vi "UpdateClassTemplate.vi"(0 "ClassWriterGOOP300In":refnum<class "ClassWriterGOOP400.lvclass">, 1 "LVClassLibraryRef":refnum<vi>, 2 "ProgressBar":refnum<vi>, 5 "error in (no error)":errorcluster) -> (14 "ClassWriterGOOP300Out":refnum<class "ClassWriterGOOP400.lvclass">, 19 "error out":errorcluster)   [LabVIEW 2020, in "ClassWriterGOOP400.lvclass"]
uses:
  <resource>/Framework/Providers/Open_GDS/ClassProviders/Provider_EndevoGOOP400/ClassWriterGOOP400_class/ClassWriterGOOP400.lvclass
  <resource>/Framework/Providers/Open_GDS/ClassProviders/Provider_LvNativeClass/ClassWriterNative_class/ClassWriterNative.lvclass
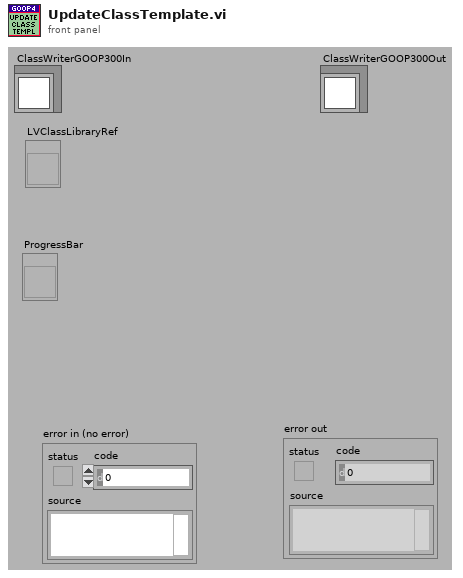
[diagram p1: front panel]
types:
  T1 = cluster{"VIs":refnum<vi>[], "VIRelPath":path[], "Application":refnum<vi>, "TemplateVersions":string, "Create":refnum<vi>, "NewVIIdx":i32, "PersistentExists":bool, "PersistentNewVersion":bool}
  T2 = enum32{"invalid lock state", "Not Locked", "Locked (No Password)", "Password-protected"}
  T3 = enum16{"Share clones between instances", "Preallocate clone for each instance"}
  T4 = typedef "GDSLvCLass_ClassSettingsType.ctl" = cluster{"ClassProviderName":string, "ClassTemplateUsed":string, "ClassTemplateVersion":string, "ClassDescription":string, "PlugIns":T5[], "ConnectorPanePattern":string}
  T5 = typedef "GDSLvClass_PlugIn.ctl" = cluster{"Type":T6, "ID":string, "Version":string, "Path":path, "Name":string, "Data":variant}
  T6 = typedef "GDSLvClass_PlugInTypes.ctl" = enum16{"DesignPattern", "MethodTypes"}
  T7 = cluster{"ID":string, "Version":string, "PlugIn":path, "Type":string, "Name":string, "Desc":string, "Supports":cluster{"Provider":string, "Templates":string}[], "DependenciesID":string[], "OnlyOne":bool}
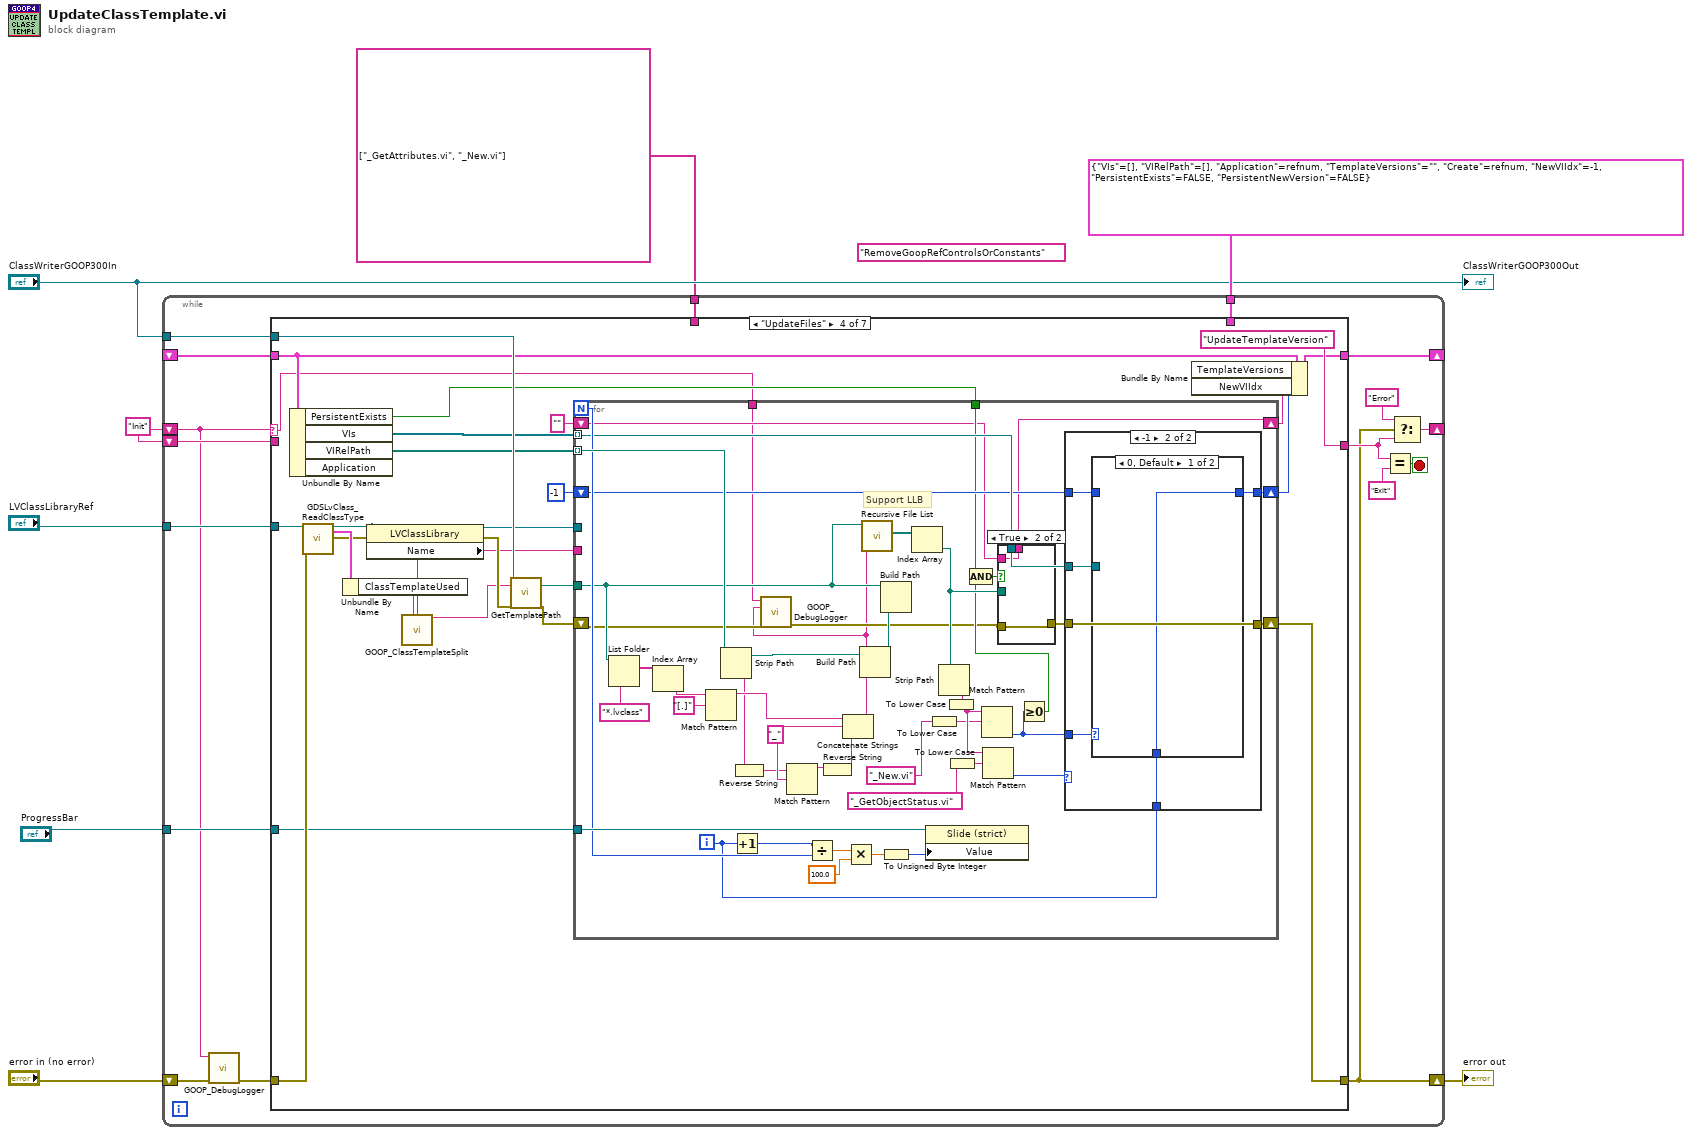
[diagram p0: block diagram]
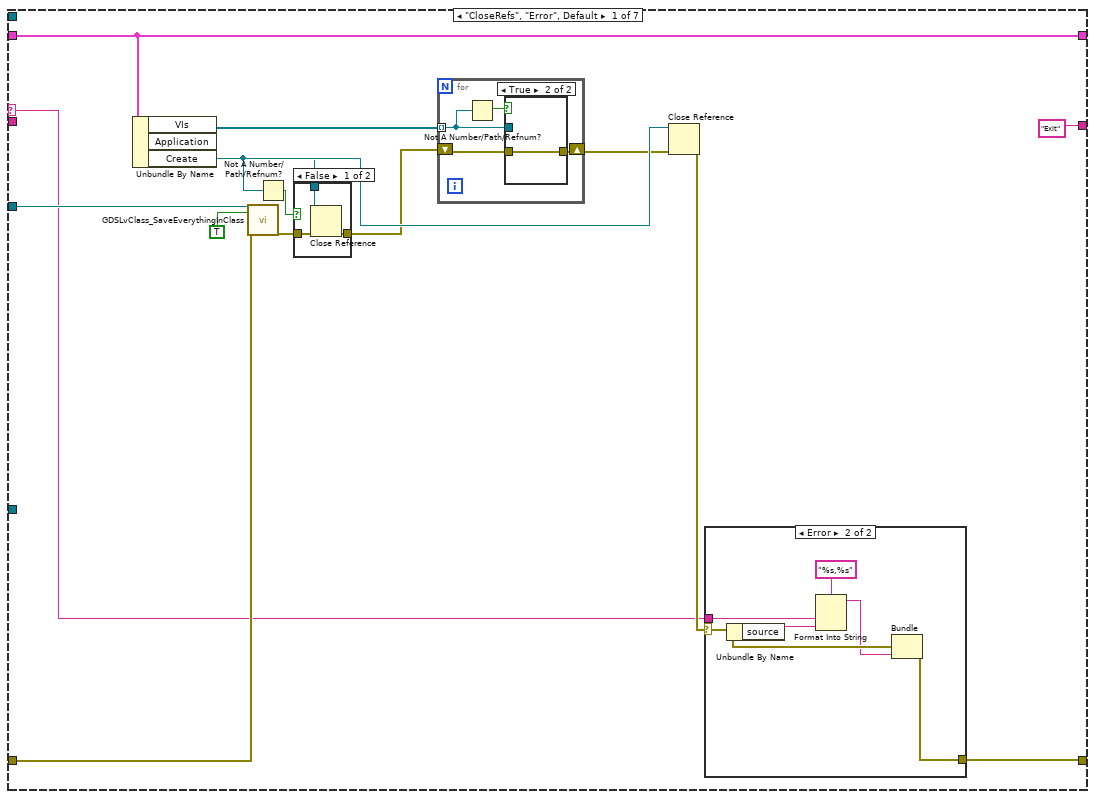
[diagram p2: hidden frame]
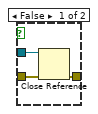
[diagram p5: hidden frame]
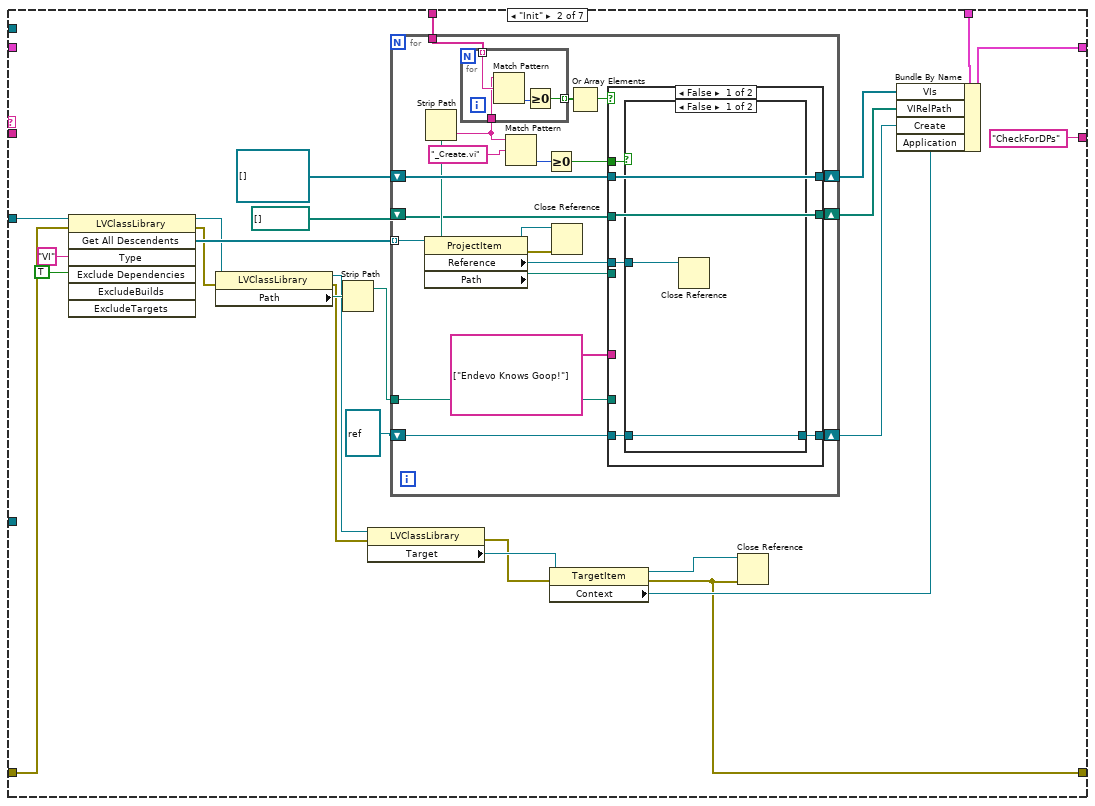
[diagram p6: hidden frame]
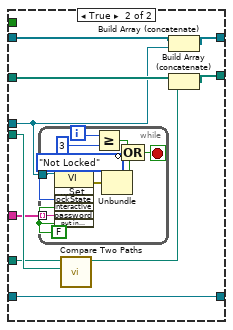
[diagram p8: hidden frame]
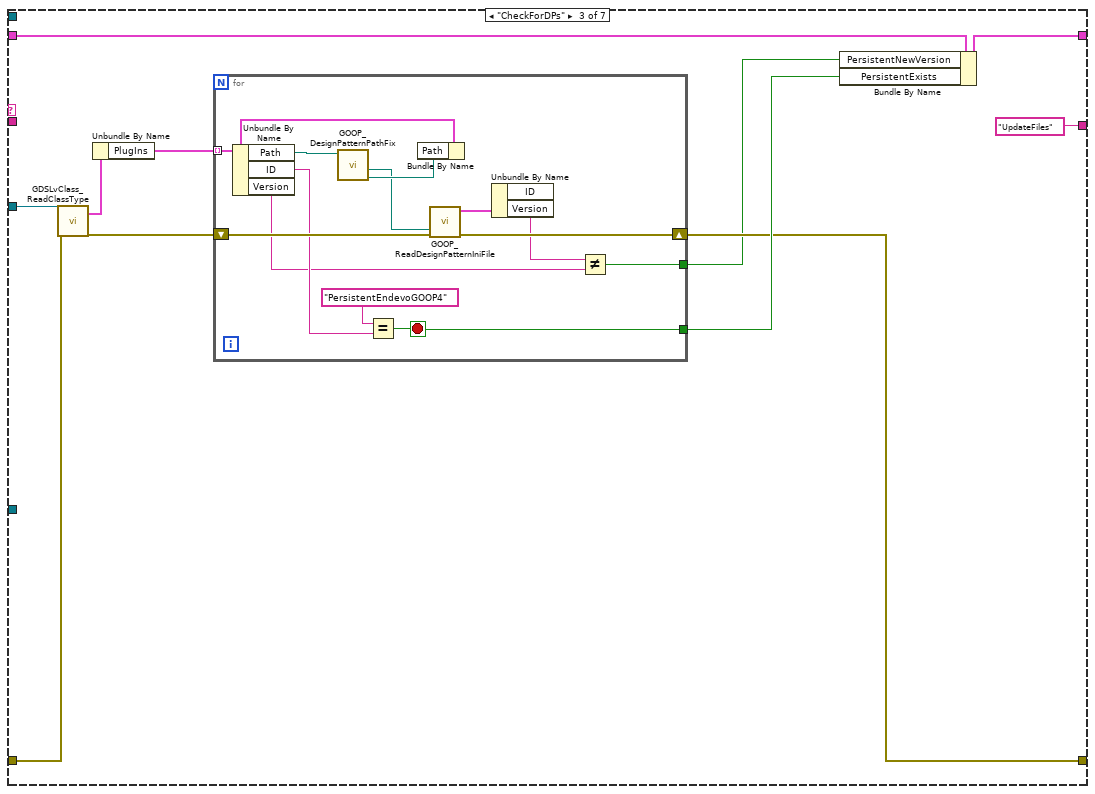
[diagram p9: hidden frame]
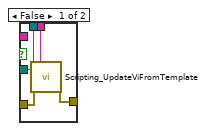
[diagram p10: hidden frame]
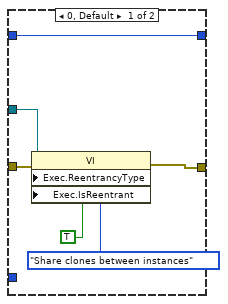
[diagram p11: hidden frame]
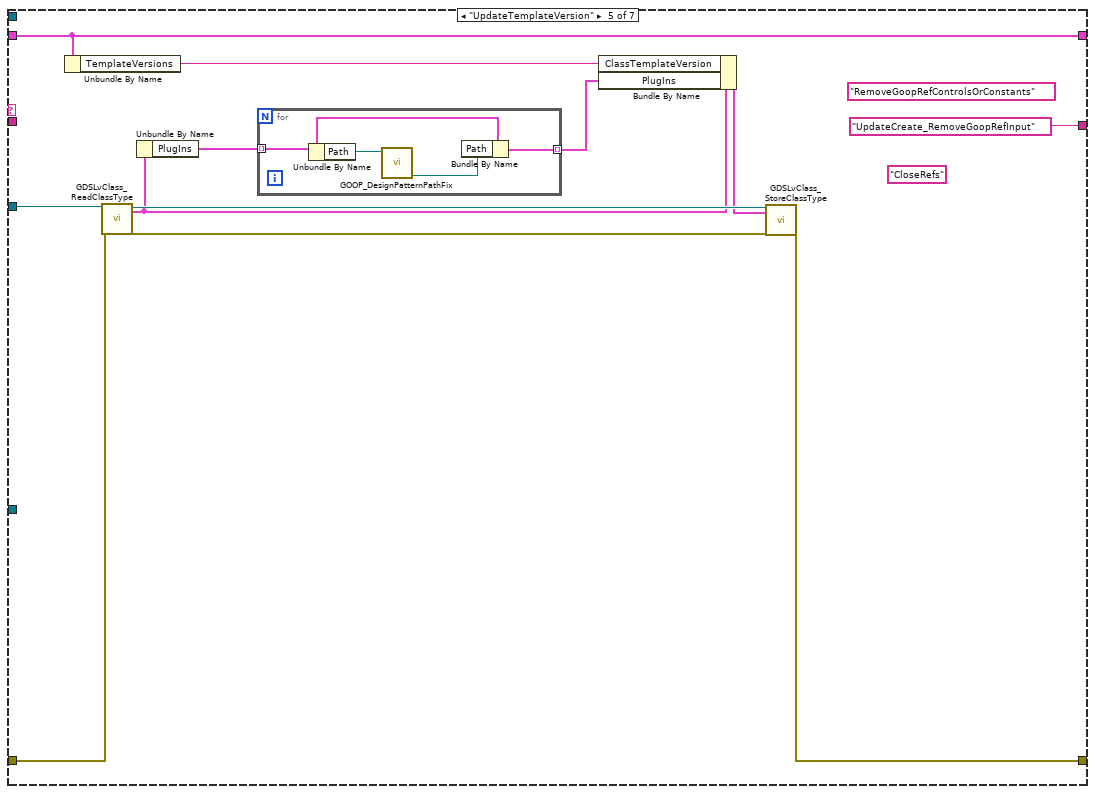
[diagram p13: hidden frame]
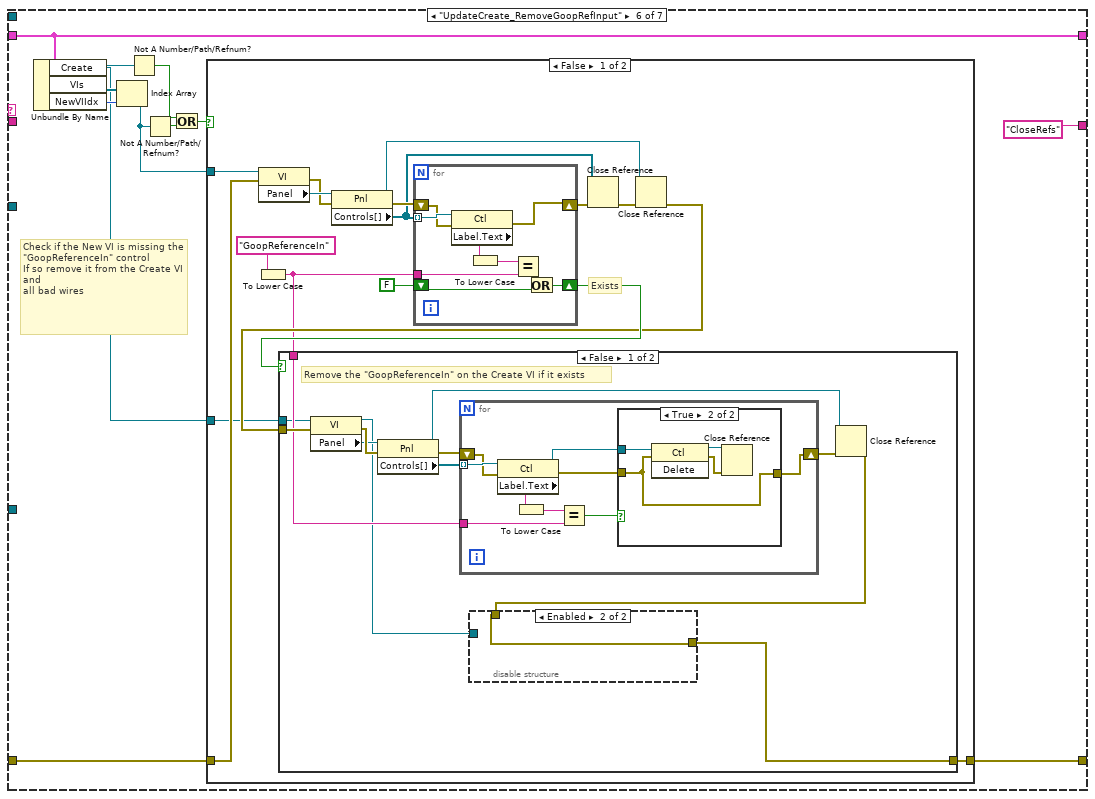
[diagram p14: hidden frame]
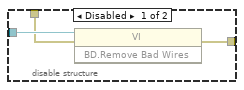
[diagram p15: hidden frame]
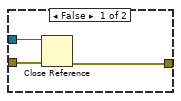
[diagram p16: hidden frame]
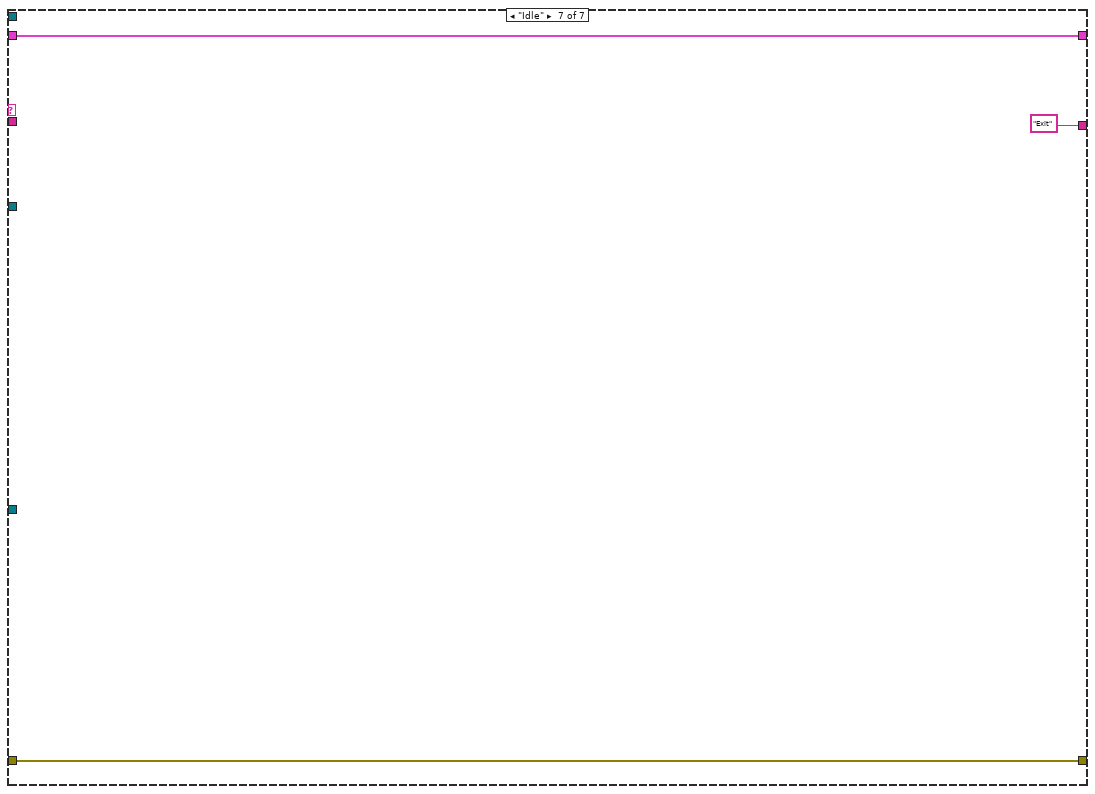
[diagram p19: hidden frame]
diagram:
  (unwired) "RemoveGoopRefControlsOrConstants"
  w1 = "Init"
  n1 = while {
    shift-right: [w20] -> w7
    shift-left: "error in (no error)" -> [w11]
    shift-right: [w25] -> _
    shift-left: w1 -> [w9]
    shift-right: [w19] -> _
    shift-left: _ -> [w18]
    tunnel: "LVClassLibraryRef" -> [w17]
    tunnel: T1 {"VIs"=[], "VIRelPath"=[], "Application"=refnum, "TemplateVersions"="", "Create"=refnum, "NewVIIdx"=-1, "PersistentExists"=FALSE, "PersistentNewVersion"=FALSE} -> [w16]
    tunnel: "ClassWriterGOOP300In" -> [w15]
    tunnel: "ProgressBar" -> [w14]
    tunnel: string[] ["_GetAttributes.vi", "_New.vi"] ("Array") -> [w13]
    shift-left: w1 -> [w12]
    stop <- w24 stop-if-true
    n2 = call <resource>:"GOOP_DebugLogger.vi"("error in (no error)"=w11, "State"=w9) -> ("error out"=w10:errorcluster)  [unwired: 7 in, 2 out]
    n3 = case shown="\"UpdateFiles\"" w9 {
      selector: w9 -> [w28 _ _ w166 _ _ _]
      tunnel: w10 -> [w34 w66 w147 w180 w261 w274 w343]
      tunnel: [w27 w61 w141 w174 w260 w273 w343] -> w20
      tunnel: ["Exit" "CheckForDPs" "UpdateFiles" "UpdateTemplateVersion" "UpdateCreate_RemoveGoopRefInput" "CloseRefs" "Exit"] -> w21
      tunnel: [w39 w85 w143 w175 w265 w280 w342] -> w19
      tunnel: w18 -> [w39 _ w139 w176 w265 w280 w342]
      tunnel: w17 -> [w35 w84 w145 w187 w264 _ _]
      tunnel: w16 -> [_ w78 _ _ _ _ _]
      tunnel: w15 -> [_ _ _ w185 _ _ _]
      tunnel: w14 -> [_ _ _ w173 _ _ _]
      tunnel: w13 -> [_ w65 _ _ _ _ _]
      tunnel: w12 -> [_ _ _ _ _ _ _]
      frame "CloseRefs", "Error", Default {
        n4 = Unbundle By Name(w39) -> ("VIs"=w38:refnum<vi>[], "Application"=w37:refnum<vi>, "Create"=w31:refnum<vi>)
        n5 = call <resource>:"GDSLvClass_SaveEverythingInClass.vi"("ClassRefIn"=w35, "ForceResaving(False)"=TRUE, "error in"=w34) -> ("error out"=w33:errorcluster)  [unwired: 15 in, 1 out]
        n6 = Not A Number/Path/Refnum?(number/path/refnum=w31) -> (NaN/Path/Refnum?=w30:bool)
        n7 = case shown="False" w30 {
          tunnel: w33 -> [w50 w51]
          tunnel: [w49 w51] -> w32
          tunnel: w31 -> [w48 _]
          frame False {
            n8 = Close Reference(reference=w48, error in (no error)=w50) -> (error out=w49:errorcluster)
          }
          frame True {
          }
        }
        n9 = for {
          tunnel: w38 -> [w53] mode=indexing
          shift-right: [w54] -> w26
          shift-left: w32 -> [w55]
          n10 = Not A Number/Path/Refnum?(number/path/refnum=w53) -> (NaN/Path/Refnum?=w52:bool)
          n11 = case shown="True" w52 {
            tunnel: w55 -> [w58 w59]
            tunnel: [w57 w59] -> w54
            tunnel: w53 -> [w56 _]
            frame False {
              n12 = Close Reference(reference=w56, error in (no error)=w58) -> (error out=w57:errorcluster)
            }
            frame True {
            }
          }
        }
        n13 = Close Reference(reference=w37, error in (no error)=w26) -> (error out=w29:errorcluster)
        n14 = case shown="Error" w29 {
          selector: w29 -> [w41 w44]
          tunnel: w28 -> [_ w46]
          tunnel: [w41 w42] -> w27
          frame No Error {
          }
          frame Error {
            n15 = Unbundle By Name(w44) -> ("source"=w45:string)
            n16 = Format Into String(format string="%s,%s", w46, w45) -> (resulting string=w43:string)  [unwired: 2 in, 1 out]
            n17 = Bundle(cluster=w44, "source"=w43) -> (w42:errorcluster)  [unwired: 2 in]
          }
        }
      }
      frame "Init" {
        n18 = invoke class="LVClassLibrary" method="Get All Descendents"(reference=w84, error in=w66, "Type"="VI", "Exclude Dependencies"=TRUE ("ExcludeDependencies")) -> (reference out=w80:refnum<vi>, error out=w69:errorcluster, "All Descendents"=w81:refnum<vi>[])  [unwired: 3 in, 4 out]
        n19 = property class="LVClassLibrary"(reference=w80, error in=w69) -> (reference out=w73:refnum<vi>, error out=w70:errorcluster, "Path"=w76:path)
        n20 = Strip Path(path=w76) -> (stripped path=w75:path)  [unwired: 1 out]
        n21 = property class="LVClassLibrary"(reference=w73, error in=w70) -> (error out=w71:errorcluster, "Target"=w72:refnum<vi>)  [unwired: 1 out]
        n22 = for {
          tunnel: w81 -> [w105] mode=indexing
          shift-right: [w103] -> w77
          shift-left: refnum<vi>[] [] -> [w104]
          shift-right: [w99] -> w68
          shift-left: path[] [] -> [w100]
          tunnel: w75 -> [w101]
          tunnel: w65 -> [w92]
          shift-right: [w88] -> w63
          shift-left: refnum<vi> refnum ("Reference") -> [w87]
          n23 = property class="ProjectItem"(reference=w105) -> (reference out=w96:refnum<vi>, error out=w98:errorcluster, "Reference"=w97:refnum<vi>, "Path"=w102:path)  [unwired: 1 in]
          n24 = Strip Path(path=w102) -> (name=w86:string)  [unwired: 1 out]
          n25 = for {
            tunnel: w92 -> [w109] mode=indexing
            tunnel: [w107] -> w94 mode=indexing
            tunnel: w86 -> [w106]
            n26 = Match Pattern(string=w106, regular expression=w109) -> (offset past match=w108:i32)  [unwired: 1 in, 3 out]
            n27 = Greater Or Equal To 0?(x=w108) -> (x >= 0?=w107:bool)
          }
          n28 = Match Pattern(string=w86, regular expression="_Create.vi") -> (offset past match=w90:i32)  [unwired: 1 in, 3 out]
          n29 = Greater Or Equal To 0?(x=w90) -> (x >= 0?=w89:bool)
          n30 = Close Reference(reference=w96, error in (no error)=w98) -> ()  [unwired: 1 out]
          n31 = Or Array Elements(Boolean array=w94) -> (logical OR=w93:bool)
          n32 = case shown="False" w93 {
            tunnel: w104 -> [w115 w128]
            tunnel: w97 -> [w111 w121]
            tunnel: [w115 w127] -> w103
            tunnel: w102 -> [_ w123]
            tunnel: w101 -> [_ w122]
            tunnel: w100 -> [w114 w126]
            tunnel: [w114 w125] -> w99
            tunnel: string[] ["Endevo Knows Goop!"] -> [_ w120]
            tunnel: w89 -> [w113 _]
            tunnel: [w112 w119] -> w88
            tunnel: w87 -> [w110 w119]
            frame False {
              n33 = case shown="False" w113 {
                tunnel: [w116 w118] -> w112
                tunnel: w111 -> [w117 w118]
                tunnel: w110 -> [w116 _]
                frame False {
                  n34 = Close Reference(reference=w117) -> ()  [unwired: 1 in, 1 out]
                }
                frame True {
                }
              }
            }
            frame True {
              n35 = while {
                tunnel: w121 -> [w136]
                tunnel: w120 -> [w135] mode=indexing
                i -> [w132]
                stop <- w133 stop-if-true
                w137 = FALSE ("Interactive")
                n36 = invoke class="VI" method="Lock State.Set"(reference=w136, "lockState"=T2."Not Locked" ("Lock State"), "interactive"=w137, "password"=w135, "put in Cache"=w137) -> (error out=w134:errorcluster)  [unwired: 2 in, 6 out]
                n37 = Greater Or Equal?(x=w132, y=3) -> (x >= y?=w131:bool)
                n38 = Unbundle(w134) -> ("status"=w129:bool)  [unwired: 2 out]
                n39 = Compound Arithmetic op=OR(w131, invert w129) -> (w133:bool)
              }
              n40 = call <vilib>:"Compare Two Paths.vi"("Path 2"=w123, "Path 1"=w122) -> ("Relative Path from 1 to 2"=w124:path)  [unwired: 6 in, 3 out]
              n41 = Build Array (concatenate)(w128, w121) -> (w127:refnum<vi>[])
              n42 = Build Array (concatenate)(w126, w124) -> (w125:path[])
            }
          }
        }
        n43 = property class="TargetItem"(reference=w72, error in=w71) -> (reference out=w60:refnum<vi>, error out=w61:errorcluster, "Context"=w67:refnum<vi>)
        n44 = Close Reference(reference=w60, error in (no error)=w61) -> ()  [unwired: 1 out]
        n45 = Bundle By Name(cluster=w78, "VIs"=w77, "VIRelPath"=w68, "Create"=w63, "Application"=w67) -> (w85:T1)
      }
      frame "CheckForDPs" {
        n46 = call <resource>:"GDSLvClass_ReadClassType.vi"("Class Refnum In"=w145, "error in (no error)"=w147) -> ("ClassSettings"=w148:T4, "error out"=w144:errorcluster)  [unwired: 15 in, 1 out]
        n47 = Unbundle By Name(w148) -> ("PlugIns"=w149:T5[])
        n48 = for {
          tunnel: w149 -> [w161] mode=indexing
          shift-right: [w156] -> w141
          shift-left: w144 -> [w158]
          tunnel: [w151] -> w142
          tunnel: [w150] -> w140
          stop <- w151 stop-if-true
          n49 = Unbundle By Name(w161) -> ("Path"=w162:path, "ID"=w155:string, "Version"=w152:string)
          n50 = call <resource>:"GOOP_DesignPatternPathFix.vi"("ViPathIn"=w162) -> ("RelativeVIPathOut(ToStoreInLvClass)"=w160:path, "Ini-File"=w159:path)  [unwired: 6 in, 3 out]
          n51 = Equal?(x="PersistentEndevoGOOP4", y=w155) -> (x = y?=w151:bool)
          n52 = Bundle By Name(cluster=w161, "Path"=w160) -> ()  [unwired: 1 out]
          n53 = call <resource>:"GOOP_ReadDesignPatternIniFile.vi"("error in (no error)"=w158, "Path"=w159) -> ("error out"=w156:errorcluster, "cluster"=w157:T7)  [unwired: 8 in]
          n54 = Unbundle By Name(w157) -> ("Version"=w153:string)  [unwired: 1 out]
          n55 = Not Equal?(x=w153, y=w152) -> (x != y?=w150:bool)
        }
        n56 = Bundle By Name(cluster=w139, "PersistentNewVersion"=w140, "PersistentExists"=w142) -> (w143:T1)
      }
      frame "UpdateFiles" {
        n57 = Unbundle By Name(w176) -> ("PersistentExists"=w169:bool, "VIs"=w182:refnum<vi>[], "VIRelPath"=w183:path[])  [unwired: 1 out]
        n58 = call <resource>:"GDSLvClass_ReadClassType.vi"("Class Refnum In"=w187, "error in (no error)"=w180) -> ("Class Refnum Out"=w163:refnum<vi>, "ClassSettings"=w186:T4, "error out"=w179:errorcluster)  [unwired: 15 in]
        n59 = Unbundle By Name(w186) -> ("ClassTemplateUsed"=w165:string)
        n60 = property class="LVClassLibrary"(reference=w163, error in=w179) -> (reference out=w172:refnum<vi>, error out=w178:errorcluster, "Name"=w177:string)
        n61 = call <resource>:"GOOP_ClassTemplateSplit.vi"("ClassItemRefIn"=w163, "FullClassTemplate"=w165) -> ("StandardTemplate"=w164:string)  [unwired: 12 in, 1 out]
        n62 = call-dynamic "GetTemplatePath.vi"("reference in"=w185, "ClassTemplateSubDirectory"=w164, "error in (no error)"=w178) -> ("FolderPathOut"=w184:path, "error out"=w181:errorcluster)  [unwired: 12 in, 3 out]
        n63 = for {
          N -> [w215]
          tunnel: w184 -> [w213]
          tunnel: w183 -> [w229] mode=indexing
          tunnel: w182 -> [w205] mode=indexing
          shift-right: [w206] -> w174
          shift-left: w181 -> [w192]
          tunnel: w177 -> [_]
          tunnel: w173 -> [w217]
          tunnel: w172 -> [_]
          shift-right: [w203] -> w170
          shift-left: -1 -> [w202]
          tunnel: w169 -> [w197]
          shift-right: [w194] -> w168
          shift-left: "" ("TemplateVersionUsed") -> [w193]
          tunnel: w166 -> [w189]
          i -> [w201]
          w233 = "_" ("regular expression")
          # "Support LLB"
          n64 = List Folder(path=w213, pattern="*.lvclass") -> (filenames=w225:string[])  [unwired: 2 in, 3 out]
          n65 = Index Array(array=w225) -> (element=w224:string)  [unwired: 1 in]
          n66 = Match Pattern(string=w224, regular expression="[.]") -> (before substring=w222:string)  [unwired: 1 in, 3 out]
          n67 = Strip Path(path=w229) -> (stripped path=w228:path, name=w221:string)
          n68 = Increment(x=w201) -> (x+1=w216:i32)
          n69 = Reverse String(1:w221) -> (0:w232:string)
          n70 = Match Pattern(string=w232, regular expression=w233) -> (before substring=w231:string)  [unwired: 1 in, 3 out]
          n71 = Divide(x=w216, y=w215) -> (x/y=w220:dbl)
          n72 = Reverse String(1:w231) -> (0:w230:string)
          n73 = Concatenate Strings(w222, w233, w230) -> (w190:string)
          n74 = call <resource>:"GOOP_DebugLogger.vi"("error in (no error)"=w192, "Data"=w190, "State"=w189) -> ("error out"=w191:errorcluster)  [unwired: 6 in, 2 out]
          n75 = Multiply(x=w220, y=100.0) -> (x*y=w218:dbl)
          n76 = Build Path(base path=w228, name or relative path=w190) -> (appended path=w227:path)
          n77 = call <vilib>:"Recursive File List.vi"("pattern"=w190, "Folder Path"=w213) -> ("All Files in Dir"=w212:path[])  [unwired: 5 in, 4 out]
          n78 = Build Path(base path=w213, name or relative path=w227) -> ()  [unwired: 1 out]
          n79 = To Unsigned Byte Integer(number=w218) -> (unsigned 8bit integer=w214:u8)
          n80 = Index Array(array=w212) -> (element=w211:path)  [unwired: 1 in]
          n81 = property class="Slide (strict)"(reference=w217, "Value"=w214) -> ()  [unwired: 1 in, 2 out]
          n82 = To Lower Case(string="_New.vi" ("regular expression")) -> (all lower case string=w199:string)
          n83 = Strip Path(path=w211) -> (name=w210:string)  [unwired: 1 out]
          n84 = To Lower Case(string=w210) -> (all lower case string=w204:string)
          n85 = To Lower Case(string="_GetObjectStatus.vi" ("regular expression")) -> (all lower case string=w208:string)
          n86 = Match Pattern(string=w204, regular expression=w199) -> (offset past match=w198:i32)  [unwired: 1 in, 3 out]
          n87 = Match Pattern(string=w204, regular expression=w208) -> (offset past match=w207:i32)  [unwired: 1 in, 3 out]
          n88 = Greater Or Equal To 0?(x=w198) -> (x >= 0?=w196:bool)
          n89 = Compound Arithmetic op=AND(w197, w196) -> (w195:bool)
          n90 = case shown="True" w195 {
            tunnel: w191 -> [w238 w240]
            tunnel: [w237 w239] -> w194
            tunnel: w211 -> [w236 _]
            tunnel: [w235 w240] -> w206
            tunnel: w205 -> [w234 _]
            tunnel: w193 -> [_ w239]
            frame False {
              n91 = call <resource>:"Scripting_UpdateViFromTemplate.vi"("ViRef"=w234, "TemplateVI(Path or Ref)"=w236, "error in (no error)"=w238) -> ("TemplateVersionUsed"=w237:string, "error out"=w235:errorcluster)  [unwired: 15 in]
            }
            frame True {
            }
          }
          n92 = case shown="-1" w207 {
            tunnel: w206 -> [w246 w252]
            tunnel: w205 -> [w245 w249]
            tunnel: [w242 w252] -> _
            tunnel: w198 -> [_ w251]
            tunnel: [w241 w250] -> w203
            tunnel: w202 -> [w241 w248]
            tunnel: w201 -> [_ w247]
            frame 0, Default {
              n93 = property class="VI"(reference=w245, error in=w246, "Exec.ReentrancyType"=T3."Share clones between instances" ("Execution:Reentrancy Type"), "Exec.IsReentrant"=TRUE ("Execution:Is Reentrant")) -> (error out=w242:errorcluster)  [unwired: 1 out]
            }
            frame -1 {
              n94 = case shown="0, Default" w251 {
                tunnel: [w253 w254] -> w250
                tunnel: w249 -> [_ _]
                tunnel: w248 -> [_ w254]
                tunnel: w247 -> [w253 _]
                frame 0, Default {
                }
                frame -1 {
                }
              }
            }
          }
        }
        n95 = Bundle By Name(cluster=w176, "TemplateVersions"=w168, "NewVIIdx"=w170) -> (w175:T1)
      }
      frame "UpdateTemplateVersion" {
        (unwired) "RemoveGoopRefControlsOrConstants"
        (unwired) "CloseRefs"
        n96 = Unbundle By Name(w265) -> ("TemplateVersions"=w257:string)
        n97 = call <resource>:"GDSLvClass_ReadClassType.vi"("Class Refnum In"=w264, "error in (no error)"=w261) -> ("Class Refnum Out"=w263:refnum<vi>, "ClassSettings"=w255:T4, "error out"=w262:errorcluster)  [unwired: 15 in]
        n98 = Unbundle By Name(w255) -> ("PlugIns"=w259:T5[])
        n99 = for {
          tunnel: w259 -> [w269] mode=indexing
          tunnel: [w267] -> w258 mode=indexing
          n100 = Unbundle By Name(w269) -> ("Path"=w270:path)
          n101 = call <resource>:"GOOP_DesignPatternPathFix.vi"("ViPathIn"=w270) -> ("RelativeVIPathOut(ToStoreInLvClass)"=w268:path)  [unwired: 6 in, 4 out]
          n102 = Bundle By Name(cluster=w269, "Path"=w268) -> (w267:T5)
        }
        n103 = Bundle By Name(cluster=w255, "ClassTemplateVersion"=w257, "PlugIns"=w258) -> (w256:T4)
        n104 = call <resource>:"GDSLvClass_StoreClassType.vi"("Class Refnum In"=w263, "ClassSettings"=w256, "error in (no error)"=w262) -> ("error out"=w260:errorcluster)  [unwired: 15 in, 1 out]
      }
      frame "UpdateCreate_RemoveGoopRefInput" {
        # "Check if the New VI is missing the\n\"GoopReferenceIn\" control\nIf so remove it from the Create VI and\nall bad wires"
        n105 = Unbundle By Name(w280) -> ("Create"=w271:refnum<vi>, "VIs"=w279:refnum<vi>[], "NewVIIdx"=w278:i32)
        n106 = Index Array(array=w279, index=w278) -> (element=w272:refnum<vi>)
        n107 = Not A Number/Path/Refnum?(number/path/refnum=w271) -> (NaN/Path/Refnum?=w277:bool)
        n108 = Not A Number/Path/Refnum?(number/path/refnum=w272) -> (NaN/Path/Refnum?=w276:bool)
        n109 = Or(x=w277, y=w276) -> (x .or. y?=w275:bool)
        n110 = case shown="False" w275 {
          tunnel: w274 -> [w287 w340]
          tunnel: [w283 w340] -> w273
          tunnel: w272 -> [w297 _]
          tunnel: w271 -> [w282 _]
          frame False {
            # "Exists"
            n111 = To Lower Case(string="GoopReferenceIn" ("y")) -> (all lower case string=w284:string)
            n112 = property class="VI"(reference=w297, error in=w287) -> (error out=w288:errorcluster, "Panel"=w296:refnum<vi>)  [unwired: 1 out]
            n113 = property class="Pnl"(reference=w296, error in=w288) -> (reference out=w289:refnum<vi>, error out=w293:errorcluster, "Controls[]"=w291:refnum<vi>[])
            n114 = for {
              tunnel: w291 -> [w339] mode=indexing
              tunnel: w284 -> [w336]
              shift-right: [w334] -> w286
              shift-left: FALSE -> [w333]
              shift-right: [w331] -> w292
              shift-left: w293 -> [w332]
              n115 = property class="Ctl"(reference=w339, error in=w332) -> (error out=w331:errorcluster, "Label.Text"=w338:string)  [unwired: 1 out]
              n116 = To Lower Case(string=w338) -> (all lower case string=w337:string)
              n117 = Equal?(x=w337, y=w336) -> (x = y?=w335:bool)
              n118 = Or(x=w335, y=w333) -> (x .or. y?=w334:bool)
            }
            n119 = Close Reference(reference=w291, error in (no error)=w292) -> (error out=w290:errorcluster)
            n120 = Close Reference(reference=w289, error in (no error)=w290) -> (error out=w285:errorcluster)
            n121 = case shown="False" w286 {
              tunnel: w285 -> [w304 w330]
              tunnel: w284 -> [w303 _]
              tunnel: [w299 w330] -> w283
              tunnel: w282 -> [w298 _]
              frame False {
                # "Remove the \"GoopReferenceIn\" on the Create VI if it exists"
                n122 = property class="VI"(reference=w298, error in=w304) -> (reference out=w301:refnum<vi>, error out=w309:errorcluster, "Panel"=w305:refnum<vi>)
                n123 = property class="Pnl"(reference=w305, error in=w309) -> (reference out=w308:refnum<vi>, error out=w306:errorcluster, "Controls[]"=w307:refnum<vi>[])
                n124 = for {
                  tunnel: w307 -> [w322] mode=indexing
                  tunnel: w303 -> [w319]
                  shift-right: [w314] -> w302
                  shift-left: w306 -> [w318]
                  n125 = property class="Ctl"(reference=w322, error in=w318) -> (reference out=w315:refnum<vi>, error out=w316:errorcluster, "Label.Text"=w321:string)
                  n126 = To Lower Case(string=w321) -> (all lower case string=w320:string)
                  n127 = Equal?(x=w320, y=w319) -> (x = y?=w317:bool)
                  n128 = case shown="True" w317 {
                    tunnel: w316 -> [w325 w328]
                    tunnel: w315 -> [w324 w329]
                    tunnel: [w323 w328] -> w314
                    frame False {
                      n129 = Close Reference(reference=w324, error in (no error)=w325) -> (error out=w323:errorcluster)
                    }
                    frame True {
                      n130 = invoke class="Ctl" method="Delete"(reference=w329, error in=w328) -> (reference out=w327:refnum<vi>, error out=w326:errorcluster)  [unwired: 1 in, 1 out]
                      n131 = Close Reference(reference=w327, error in (no error)=w326) -> ()  [unwired: 1 out]
                    }
                  }
                }
                n132 = Close Reference(reference=w308, error in (no error)=w302) -> (error out=w300:errorcluster)
                n133 = disable-structure shown="Enabled" {
                  disable-tunnel: w301 -> [w312 _]
                  disable-tunnel: w300 -> [w311 w313]
                  disable-tunnel: [w310 w313] -> w299
                  frame Disabled {
                    n134 = invoke class="VI" method="BD.Remove Bad Wires"(reference=w312, error in=w311) -> (error out=w310:errorcluster)  [unwired: 1 in, 2 out]
                  }
                  frame Enabled {
                  }
                }
              }
              frame True {
                # "Don't do anything"
              }
            }
          }
          frame True {
          }
        }
      }
      frame "Idle" {
      }
    }
    n135 = Equal?(x=w21, y="Exit") -> (x = y?=w24:bool)
    n136 = Select(t="Error", s=w20, f=w21) -> (s? t:f=w25:string)
  }
  "error out" <- w7
  "ClassWriterGOOP300Out" <- "ClassWriterGOOP300In"
